vi "FT10_M4X Tester 3.vi"() -> ()   [LabVIEW 2024]
uses:
  Controls/QMH Fundamentals - Message Cluster.ctl
  <vilib>/FPGAPlugInAG/PXI-7854R/niLvFpga_Open_PXI-7854R.vi
  <vilib>/rvi/interface/common/dynamic/niFpgaDynamicAddResources.vi
  <vilib>/Utility/error.llb/Error Cluster From Error Code.vi
  <vilib>/rvi/errors/niLvFpgaAdjustHostInterfaceError.vi
  <vilib>/FPGAPlugInAG/Dynamic/niLvFpga_Close_Dynamic.vi
  <vilib>/rvi/interface/nirviOpenFPGA/nirviOpenFPGA.xnode
  FPGA Bitfiles/FT10_FPGA_7854R_Main_Rev4 BitFile.lvbitx
  FT10_FPGA_7854R_Main 4.vi
  <vilib>/rvi/interface/nirviReadWriteControl/nirviReadWriteControl.xnode
  <vilib>/rvi/interface/nirviCloseFPGA/nirviCloseFPGA.xnode
  <vilib>/rvi/interface/Simulation/niFpgaSimulationCallBeginRW.vi
  spcm_win32.dll
  NiFpgaLv.dll
panel:
  in  "Update Relays":bool
  in  "Tab Control":T1(tab)
  in  "Update Config Enum":T2(ring)
  in  "Update Config":bool
  out "Connector0/AI0":i16
  out "Connector0/AI1":i16
  out "Connector0/AI2":i16
  out "Connector0/AI3":i16
  out "Connector0/AI4":i16
  out "Connector0/AI5":i16
  out "Connector0/AI6":i16
  out "Connector0/AI7":i16
  in  "Connector0/AO0":i16
  in  "Connector0/AO2":i16
  in  "Connector0/AO3":i16
  in  "Connector0/AO4":i16
  in  "Connector0/AO5":i16
  in  "Connector0/AO6":i16
  in  "Connector0/AO1":i16
  in  "Connector0/AO7":i16
  in  "Conn0/DIO_8_15 - 75kHz":bool=TRUE
  in  "Conn0/DIO_8_15 - uSec On":u16=7
  in  "Conn0/DIO_8_15 - uSec Off":u16=6
  in  "Conn0/DIO_0_7 - uSec Off":u16=6
  in  "Conn0/DIO_0_7 - uSec On":u16=7
  in  "Conn0/DIO_0_7 - 75kHz":bool=TRUE
  in  "Conn0/DIO_8_15 In":bool[](array[boolean])=[FALSE, FALSE, FALSE, FALSE, FALSE, FALSE, FALSE, FALSE]
  in  "Conn0/DIO_0_7 In":bool[](array[boolean])=[FALSE, FALSE, FALSE, FALSE, FALSE, FALSE, FALSE, FALSE]
  out "Conn0/DIO_0_7 Out":bool[](array[boolean])
  out "Conn0/DIO_8_15 Out":bool[](array[boolean])
  in  "Conn1/DIO_32_39 - 75kHz":bool=TRUE
  in  "Conn1/DIO_32_39 - uSec On":u16=7
  in  "Conn1/DIO_32_39 - uSec Off":u16=6
  in  "Conn1/DIO_32_39 In":bool[](array[boolean])=[FALSE, FALSE, FALSE, FALSE, FALSE, FALSE, FALSE, FALSE]
  out "Conn1/DIO_32_39 Out":bool[](array[boolean])
  in  "Conn1/DIO_24_31 - 75kHz":bool=TRUE
  in  "Conn1/DIO_24_31 - uSec On":u16=7
  in  "Conn1/DIO_24_31 - uSec Off":u16=6
  in  "Conn1/DIO_16_23 - uSec Off":u16=6
  in  "Conn1/DIO_16_23 - uSec On":u16=7
  in  "Conn1/DIO_16_23 - 75kHz":bool=TRUE
  in  "Conn1/DIO_24_31 In":bool[](array[boolean])=[FALSE, FALSE, FALSE, FALSE, FALSE, FALSE, FALSE, FALSE]
  in  "Conn1/DIO_16_23 In":bool[](array[boolean])=[FALSE, FALSE, FALSE, FALSE, FALSE, FALSE, FALSE, FALSE]
  out "Conn1/DIO_16_23 Out":bool[](array[boolean])
  out "Conn1/DIO_24_31 Out":bool[](array[boolean])
  in  "Conn1/DIO_8_15 - 75kHz":bool=TRUE
  in  "Conn1/DIO_8_15 - uSec On":u16=7
  in  "Conn1/DIO_8_15 - uSec Off":u16=6
  in  "Conn1/DIO_0_7 - uSec Off":u16=6
  in  "Conn1/DIO_0_7 - uSec On":u16=7
  in  "Conn1/DIO_0_7 - 75kHz":bool=TRUE
  in  "Conn1/DIO_8_15 In":bool[](array[boolean])=[FALSE, FALSE, FALSE, FALSE, FALSE, FALSE, FALSE, FALSE]
  in  "Conn1/DIO_0_7 In":bool[](array[boolean])=[FALSE, FALSE, FALSE, FALSE, FALSE, FALSE, FALSE, FALSE]
  out "Conn1/DIO_0_7 Out":bool[](array[boolean])
  out "Conn1/DIO_8_15 Out":bool[](array[boolean])
  in  "Conn2/DIO_32_39 - 75kHz":bool=TRUE
  in  "Conn2/DIO_32_39 - uSec On":u16=7
  in  "Conn2/DIO_32_39 - uSec Off":u16=6
  in  "Conn2/DIO_32_39 In":bool[](array[boolean])=[FALSE, FALSE, FALSE, FALSE, FALSE, FALSE, FALSE, FALSE]
  out "Conn2 /DIO_32_39 Out":bool[](array[boolean])
  in  "Conn2/DIO_24_31 - 75kHz":bool=TRUE
  in  "Conn2/DIO_24_31 - uSec On":u16=7
  in  "Conn2/DIO_24_31 - uSec Off":u16=6
  in  "Conn2/DIO_16_23 - uSec Off":u16=6
  in  "Conn2/DIO_16_23 - uSec On":u16=7
  in  "Conn2/DIO_16_23 - 75kHz":bool=TRUE
  in  "Conn2/DIO_24_31 In":bool[](array[boolean])=[FALSE, FALSE, FALSE, FALSE, FALSE, FALSE, FALSE, FALSE]
  in  "Conn2/DIO_16_23 In":bool[](array[boolean])=[FALSE, FALSE, FALSE, FALSE, FALSE, FALSE, FALSE, FALSE]
  out "Conn2/DIO_16_23 Out":bool[](array[boolean])
  out "Conn2/DIO_24_31 Out":bool[](array[boolean])
  in  "Conn2/DIO_8_15 - 75kHz":bool=TRUE
  in  "Conn2/DIO_8_15 - uSec On":u16=7
  in  "Conn2/DIO_8_15 - uSec Off":u16=6
  in  "Conn2/DIO_0_7 - uSec Off":u16=6
  in  "Conn2/DIO_0_7 - uSec On":u16=7
  in  "Conn2/DIO_0_7 - 75kHz":bool=TRUE
  in  "Conn2/DIO_8_15 In":bool[](array[boolean])=[FALSE, FALSE, FALSE, FALSE, FALSE, FALSE, FALSE, FALSE]
  in  "Conn2/DIO_0_7 In":bool[](array[boolean])=[FALSE, FALSE, FALSE, FALSE, FALSE, FALSE, FALSE, FALSE]
  out "Conn2/DIO_0_7 Out":bool[](array[boolean])
  out "Conn2/DIO_8_15 Out":bool[](array[boolean])
  out "error out 2":errorcluster
  out "error out":errorcluster
  out "Array":T3(array[cluster])
  out "Waveform Array":waveform(dbl)[](graph)
  in  "stop":bool
  in  "Read":bool
  # "Conn0/DIO_0_7"
  # "Conn0/DIO_8_15"
  # "Conn0/AO_0_7"
  # "Conn0/AI0_7"
  # "Conn1/DIO_0_7"
  # "Conn1/DIO_8_15"
  # "Conn1/DIO_16_23"
  # "Conn1/DIO_24_31"
  # "Conn1/DIO_32_39"
  # "Conn2/DIO_0_7"
  # "Conn2/DIO_8_15"
  # "Conn2/DIO_16_23"
  # "Conn2/DIO_24_31"
  # "Conn2/DIO_32_39"
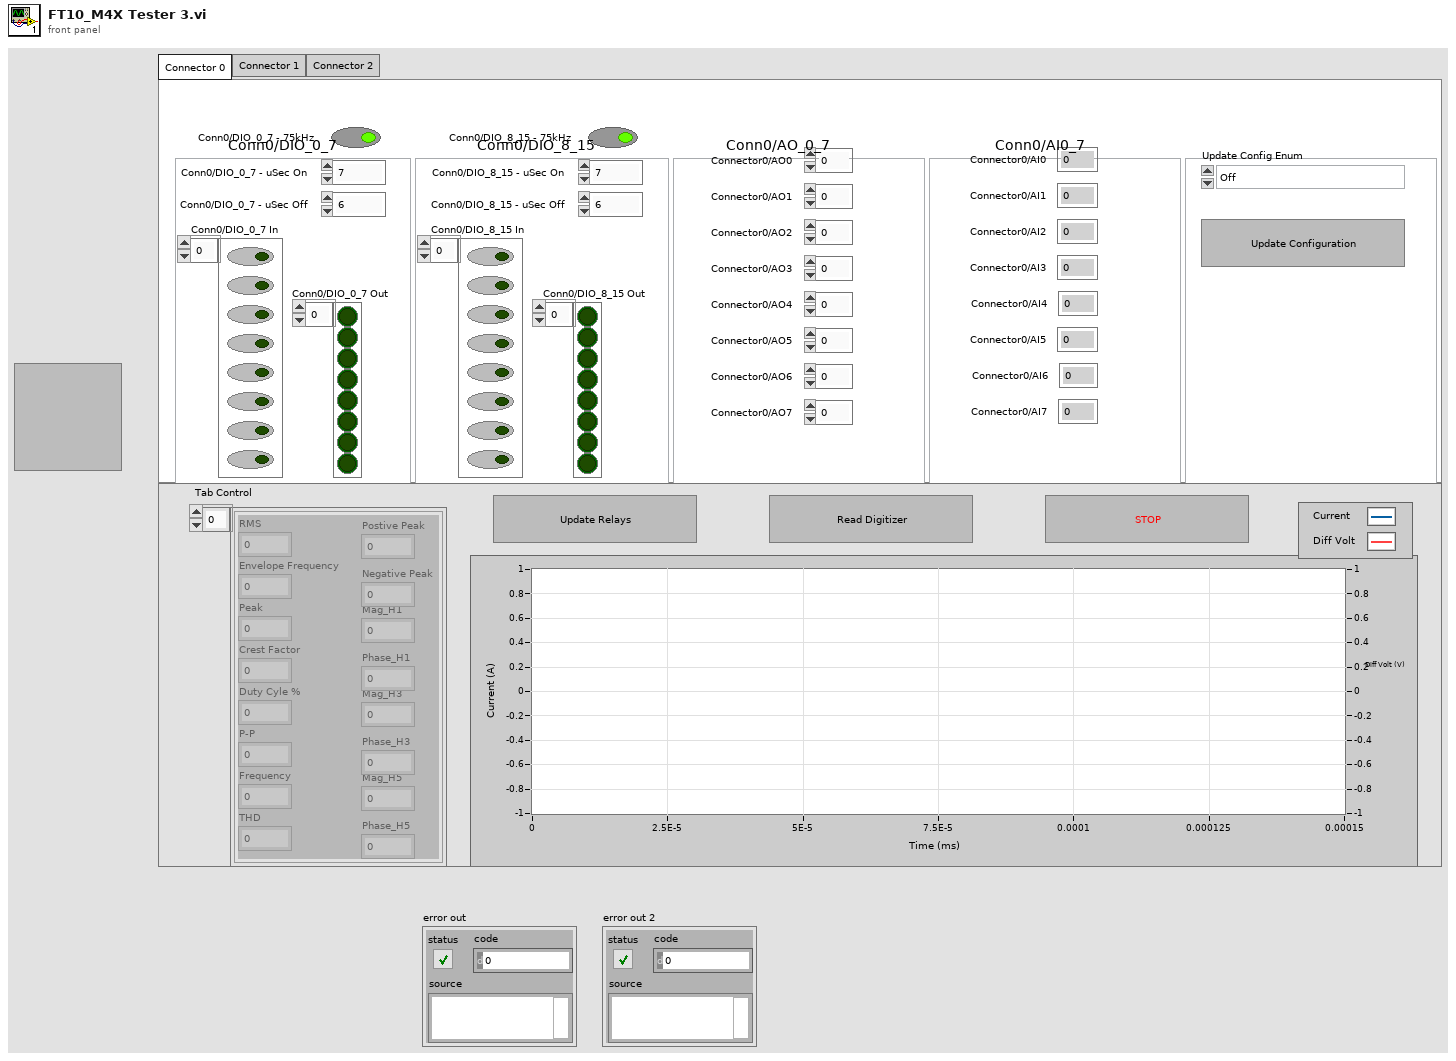
[diagram p1: front panel]
types:
  T1 = enum32{"Connector 0", "Connector 1", "Connector 2"}
  T2 = enum16{"Off", "Mono1 Relay Config", "Mono2 Relay Config", "Bipolar Relay Config", "Ligasure Relay Config", "Handswitch - Mono1 Cut", "Handswitch - Mono1 Coag", "Handswitch - Mono2 Cut", "Handswitch - Mono2 Coag", "Switch to Triverse Mode", "Switch to Mono2 - 2 button Mode", "Triverse Power 1", "Triverse Power 2", "Triverse Power 3", "Triverse Power 4", "Triverse Power 5", "Handswitch - Triverse Seal", "Handswitch - Triverse Cut", "Handswitch - Triverse Coag"}
  T3 = cluster{"RMS":dbl, "Envelope Frequency":dbl, "Peak":dbl, "Crest Factor":dbl, "Duty Cyle %":dbl, "P-P":dbl, "Frequency":dbl, "THD":dbl, "Postive Peak":dbl, "Negative Peak":dbl, "Mag_H1":dbl, "Phase_H1":dbl, "Mag_H3":dbl, "Phase_H3":dbl, "Mag_H5":dbl, "Phase_H5":dbl}[]
  T4 = typedef "QMH Fundamentals - Message Cluster.ctl" = cluster{"Message":string, "Message Data":variant}
  T5 = cluster{"Conn1/DIO_0_7 In":cluster{"Conn1/DIO_0_7 - 75kHz":bool, "Conn1/DIO_0_7 - uSec On":u16, "Conn1/DIO_0_7 In":bool[], "Conn1/DIO_0_7 - uSec Off":u16}, "Conn1/DIO_8_15 In":cluster{"Conn1/DIO_8_15 - 75kHz":bool, "Conn1/DIO_8_15 - uSec On":u16, "Conn1/DIO_8_15 In":bool[], "Conn1/DIO_8_15 - uSec Off":u16}, "Conn1/DIO_16_23 In":cluster{"Conn1/DIO_16_23 - 75kHz":bool, "Conn1/DIO_16_23 - uSec On":u16, "Conn1/DIO_16_23 In":bool[], "Conn1/DIO_16_23 - uSec Off":u16}, "Conn1/DIO_24_31 In":cluster{"Conn1/DIO_24_31 - 75kHz":bool, "Conn1/DIO_24_31 - uSec On":u16, "Conn1/DIO_24_31 In":bool[], "Conn1/DIO_24_31 - uSec Off":u16}, "Conn1/DIO_32_39 In":cluster{"Conn1/DIO_32_39 - 75kHz":bool, "Conn1/DIO_32_39 - uSec On":u16, "Conn1/DIO_32_39 In":bool[], "Conn1/DIO_32_39 - uSec Off":u16}}
  T6 = cluster{"Conn0/DIO_0_7 In":cluster{"Conn0/DIO_0_7 - 75kHz":bool, "Conn0/DIO_0_7 - uSec On":u16, "Conn0/DIO_0_7 In":bool[], "Conn0/DIO_0_7 - uSec Off":u16}, "Conn0/DIO_8_15 In":cluster{"Conn0/DIO_8_15 - 75kHz":bool, "Conn0/DIO_8_15 - uSec On":u16, "Conn0/DIO_8_15 In":bool[], "Conn0/DIO_8_15 - uSec Off":u16}}
  T7 = cluster{"Update Config":bool, "Update Config Enum":enum16{"Off", "Mono1 Relay Config", "Mono2 Relay Config", "Bipolar Relay Config", "Ligasure Relay Config", "Handswitch - Mono1 Cut", "Handswitch - Mono1 Coag", "Handswitch - Mono2 Cut", "Handswitch - Mono2 Coag", "Switch to Triverse Mode", "Switch to Mono2 - 2 button Mode", "Triverse Power 1", "Triverse Power 2", "Triverse Power 3", "Triverse Power 4", "Triverse Power 5", "Handswitch - Triverse Seal", "Handswitch - Triverse Cut", "Handswitch - Triverse Coag"}}
  T8 = cluster{"RMS":dbl, "Envelope Frequency":dbl, "Peak":dbl, "Crest Factor":dbl, "Duty Cyle %":dbl, "P-P":dbl, "Frequency":dbl, "THD":dbl, "Postive Peak":dbl, "Negative Peak":dbl, "Mag_H1":dbl, "Phase_H1":dbl, "Mag_H3":dbl, "Phase_H3":dbl, "Mag_H5":dbl, "Phase_H5":dbl}
  T9 = cluster{"Conn2/DIO_0_7 In":cluster{"Conn2/DIO_0_7 - 75kHz":bool, "Conn2/DIO_0_7 - uSec On":u16, "Conn2/DIO_0_7 In":bool[], "Conn2/DIO_0_7 - uSec Off":u16}, "Conn2/DIO_8_15 In":cluster{"Conn2/DIO_8_15 - 75kHz":bool, "Conn2/DIO_8_15 - uSec On":u16, "Conn2/DIO_8_15 In":bool[], "Conn2/DIO_8_15 - uSec Off":u16}, "Conn2/DIO_16_23 In":cluster{"Conn2/DIO_16_23 - 75kHz":bool, "Conn2/DIO_16_23 - uSec On":u16, "Conn2/DIO_16_23 In":bool[], "Conn2/DIO_16_23 - uSec Off":u16}, "Conn2/DIO_24_31 In":cluster{"Conn2/DIO_24_31 - 75kHz":bool, "Conn2/DIO_24_31 - uSec On":u16, "Conn2/DIO_24_31 In":bool[], "Conn2/DIO_24_31 - uSec Off":u16}, "Conn2/DIO_32_39 In":cluster{"Conn2/DIO_32_39 - 75kHz":bool, "Conn2/DIO_32_39 - uSec On":u16, "Conn2/DIO_32_39 In":bool[], "Conn2/DIO_32_39 - uSec Off":u16}}
  T10 = cluster{"Conn0/DIO_0_7 Out":bool[], "Conn0/DIO_8_15 Out":bool[]}
  T11 = cluster{"Conn1/DIO_0_7 Out":bool[], "Conn1/DIO_8_15 Out":bool[], "Conn1/DIO_16_23 Out":bool[], "Conn1/DIO_24_31 Out":bool[], "Conn1/DIO_32_39 Out":bool[]}
  T12 = cluster{"Conn2/DIO_0_7 Out":bool[], "Conn2/DIO_8_15 Out":bool[], "Conn2/DIO_16_23 Out":bool[], "Conn2/DIO_24_31 Out":bool[], "Conn2/DIO_32_39 Out":bool[]}
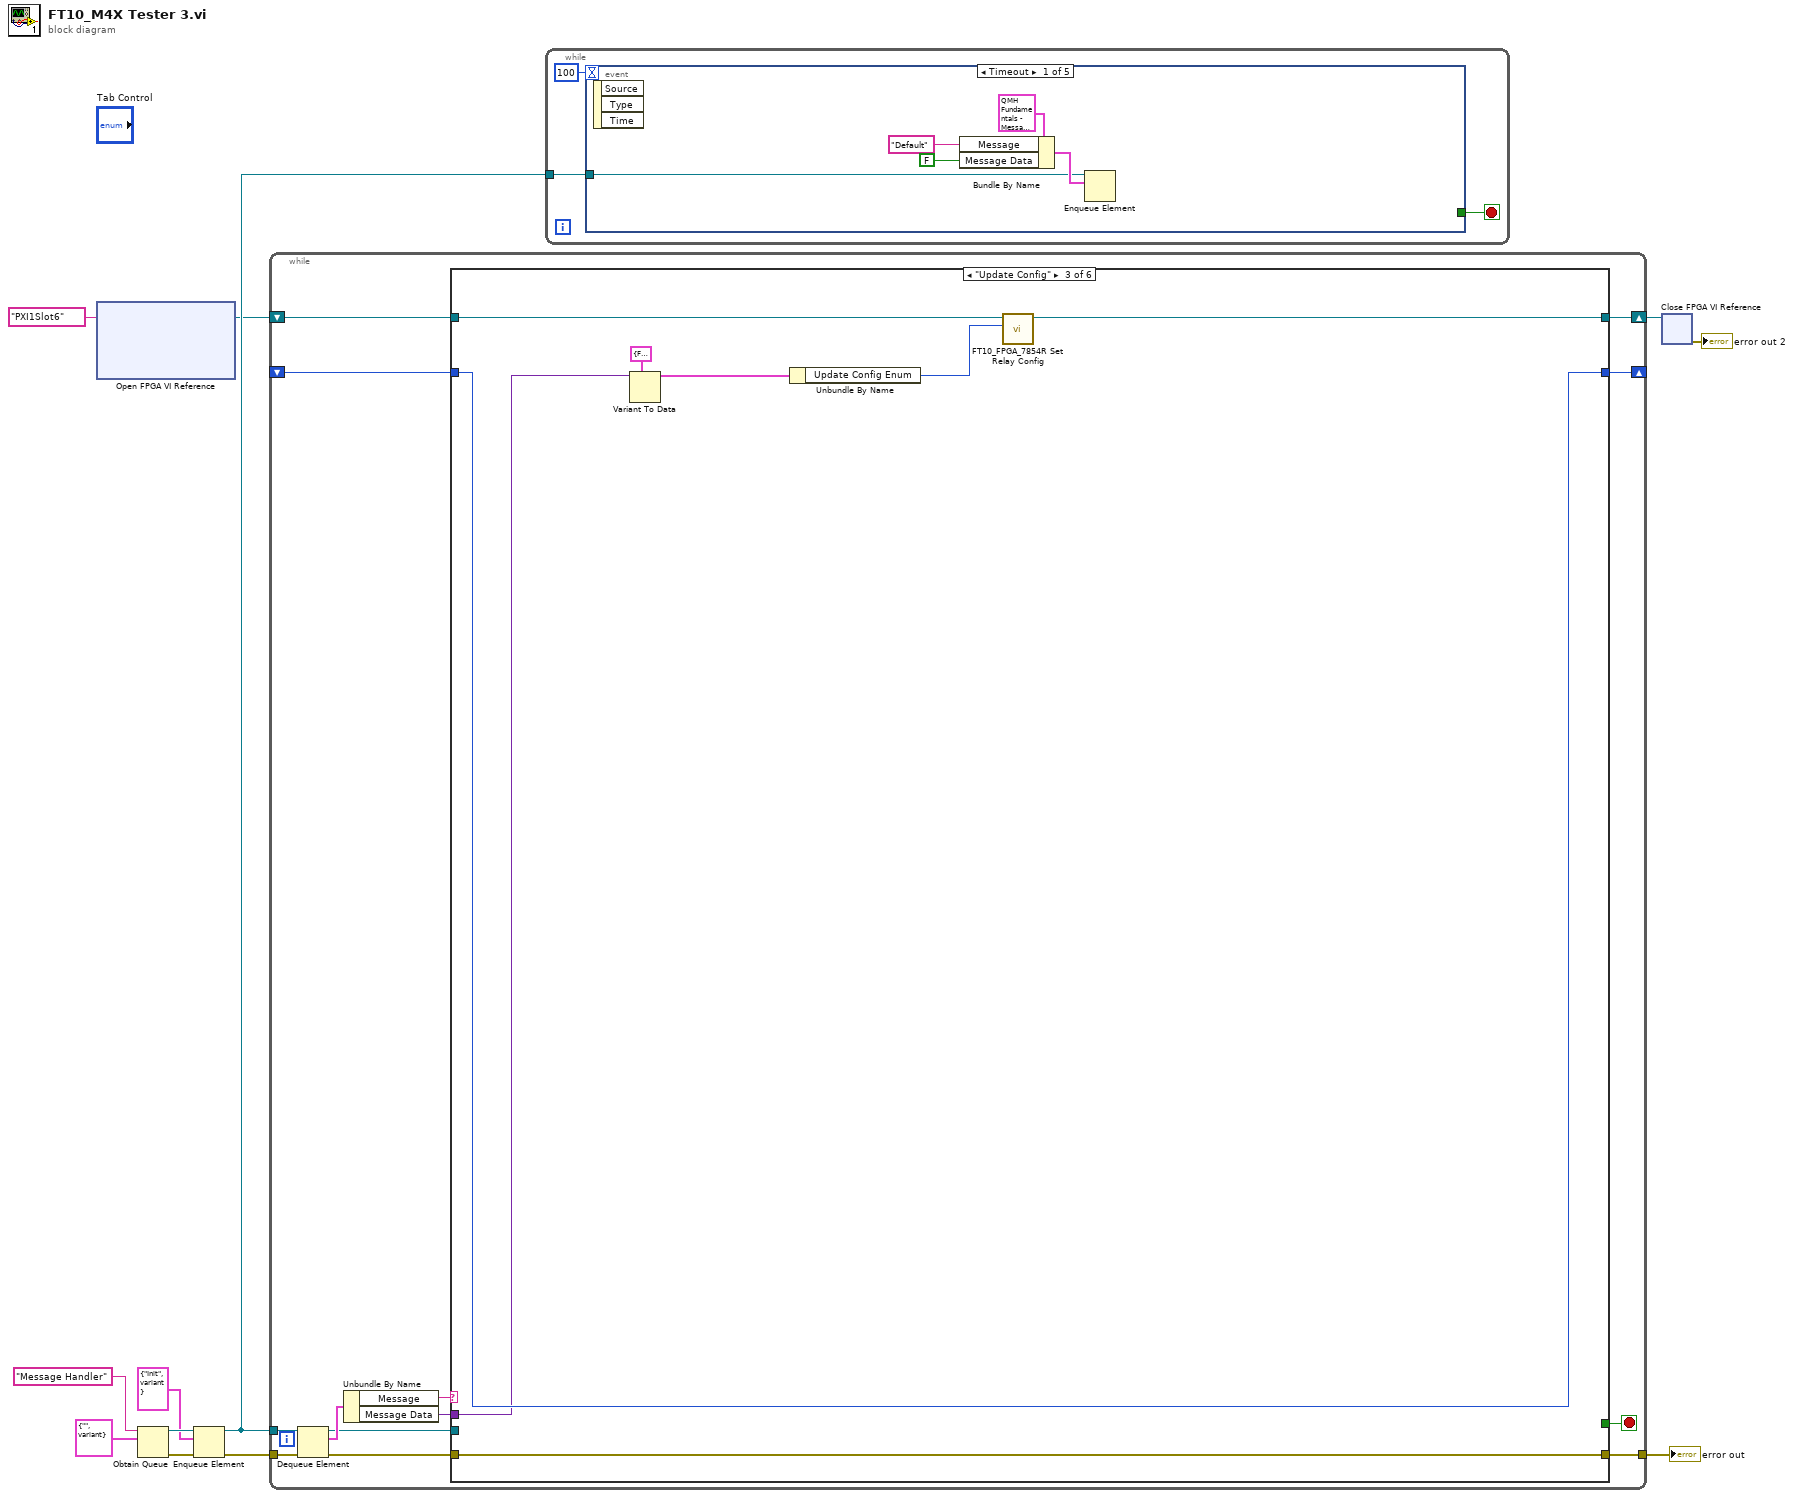
[diagram p0: block diagram]
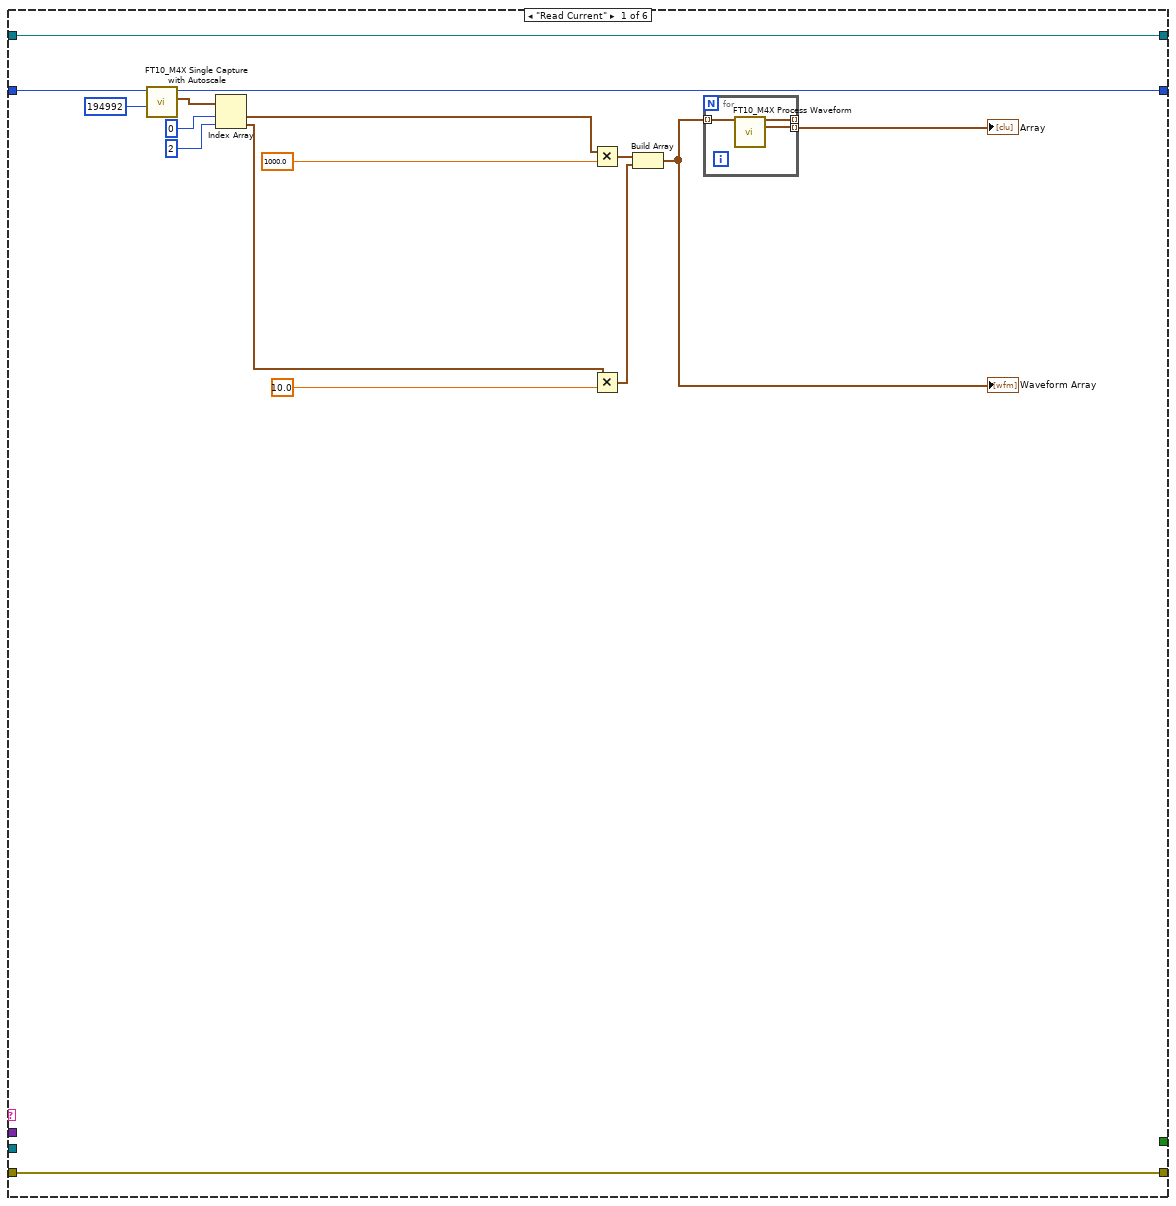
[diagram p2: hidden frame]
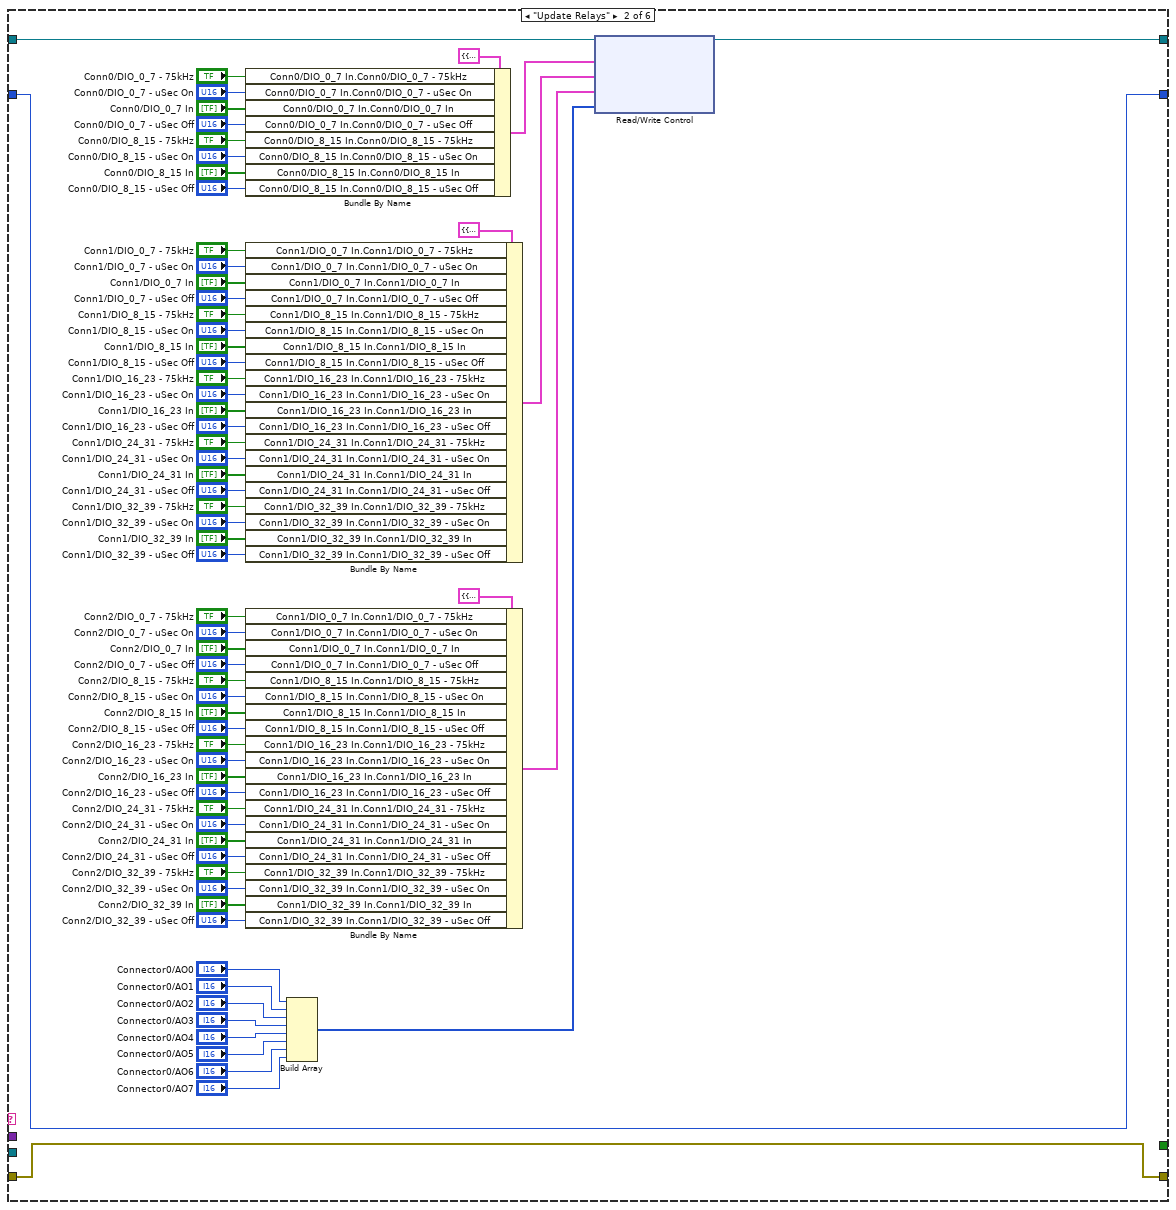
[diagram p3: hidden frame]
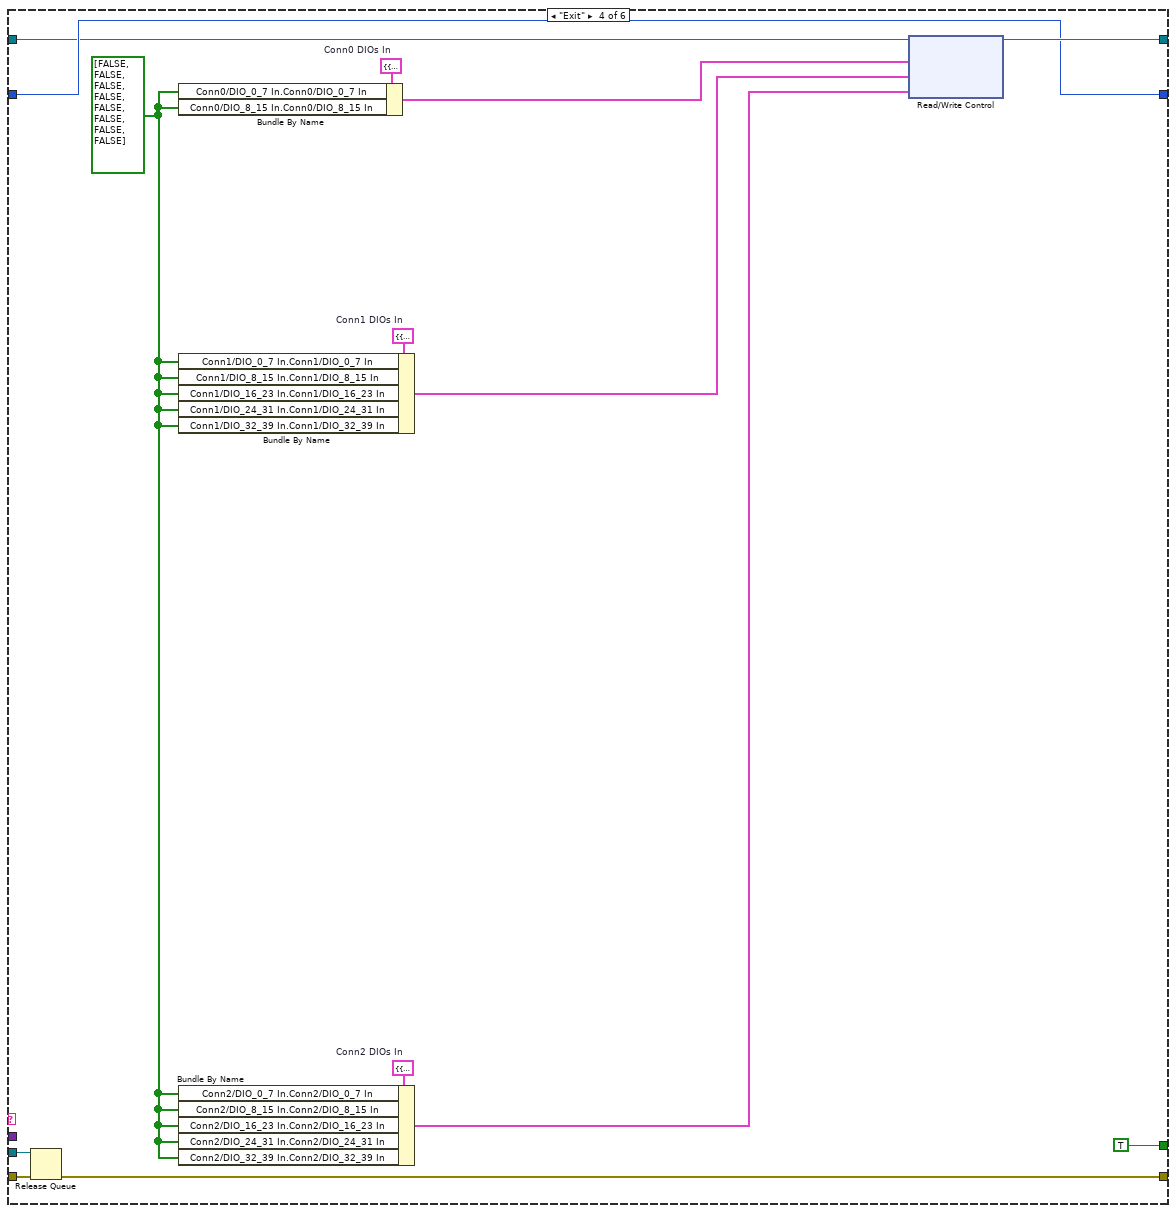
[diagram p4: hidden frame]
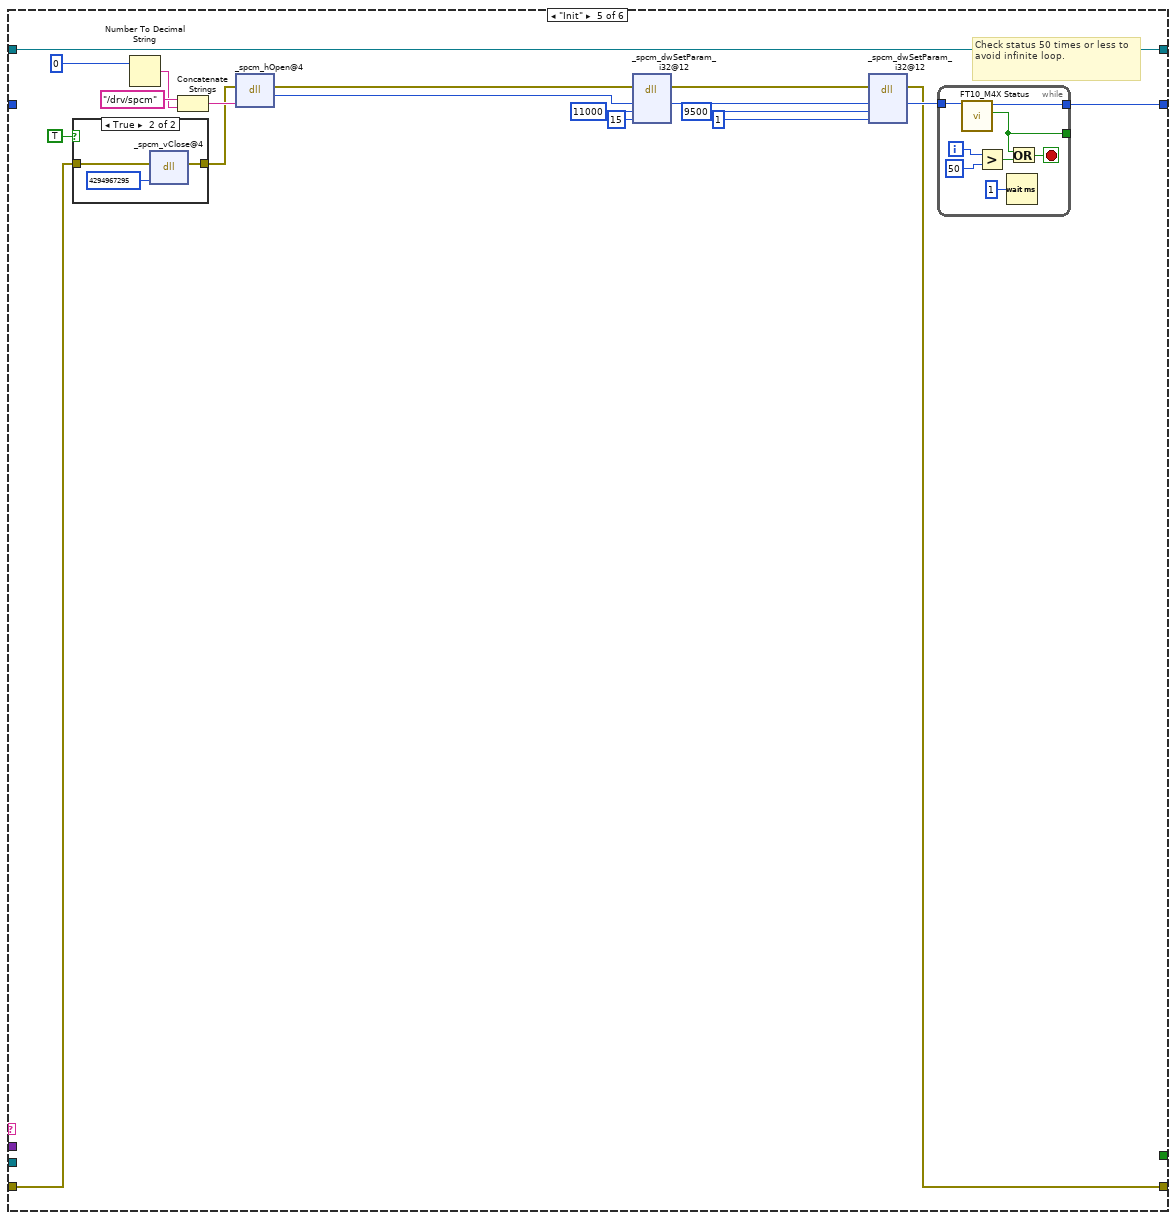
[diagram p5: hidden frame]
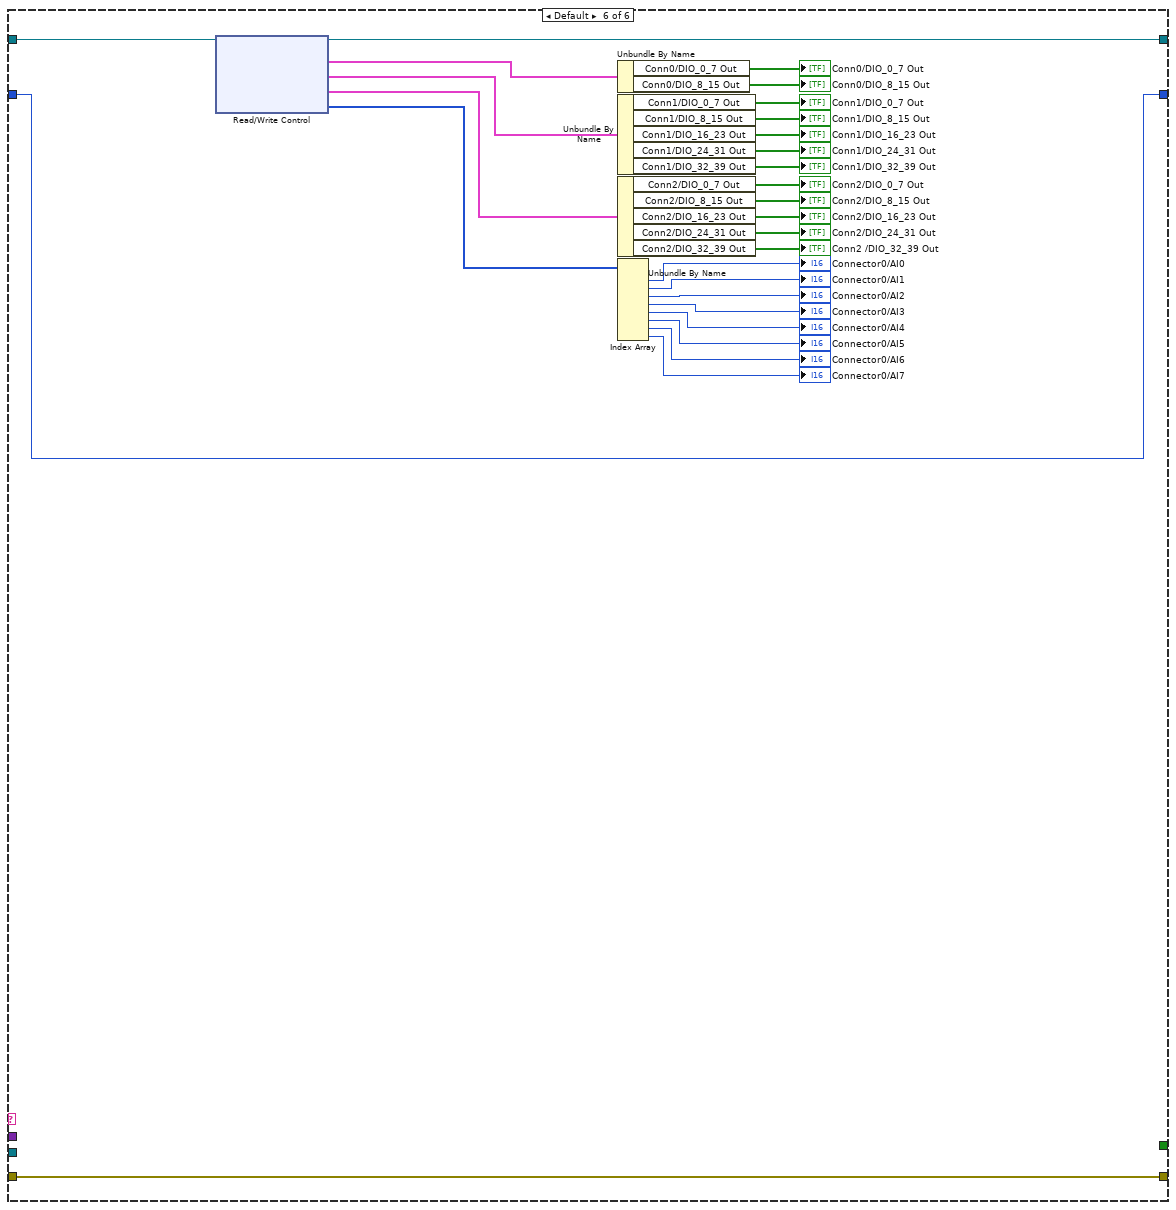
[diagram p7: hidden frame]
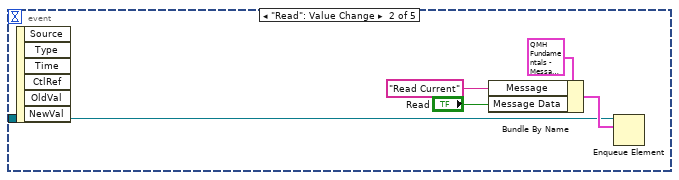
[diagram p8: hidden frame]
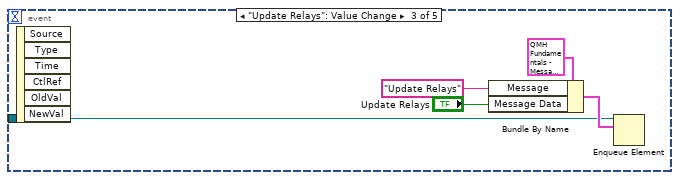
[diagram p9: hidden frame]
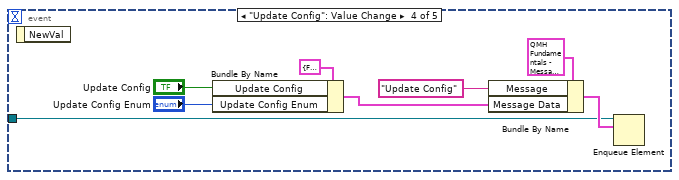
[diagram p10: hidden frame]
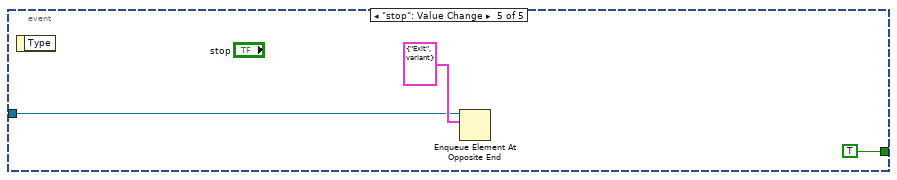
[diagram p11: hidden frame]
diagram:
  n1 = xnode "Open FPGA VI Reference"("resource name"=tag "PXI1Slot6") -> ("FPGA VI Reference Out"=w1:refnum<k20>)  [unwired: 1 in, 1 out]
  n2 = Obtain Queue(name (unnamed)="Message Handler", element data type=T4 {"Message"="", "Message Data"=variant} ("Message Cluster")) -> (queue out=w10:refnum<queue>, error out=w11:errorcluster)  [unwired: 3 in, 1 out]
  n3 = Enqueue Element(queue=w10, element=T4 {"Message"="Init", "Message Data"=variant}, error in (no error)=w11) -> (queue out=w5:refnum<queue>, error out=w7:errorcluster)  [unwired: 1 in, 1 out]
  n4 = while {
    tunnel: w5 -> [w24]
    tunnel: w7 -> [w23]
    tunnel: [w18] -> w6
    shift-right: [w17] -> _
    shift-left: _ -> [w16]
    shift-right: [w14] -> w4
    shift-left: w1 -> [w13]
    stop <- w15 stop-if-true
    n5 = Dequeue Element(queue=w24, error in (no error)=w23) -> (queue out=w22:refnum<queue>, element=w25:T4, error out=w21:errorcluster)  [unwired: 1 in, 1 out]
    n6 = Unbundle By Name(w25) -> ("Message"=w20:string, "Message Data"=w19:variant)
    n7 = case shown="\"Update Config\"" w20 {
      tunnel: w22 -> [_ _ _ w130 _ _]
      tunnel: w21 -> [w30 w108 w116 w132 w137 w192]
      tunnel: w19 -> [_ _ w114 _ _ _]
      tunnel: [w30 w108 w116 w131 w136 w192] -> w18
      tunnel: [w31 w109 w117 w128 w135 w189] -> w17
      tunnel: w16 -> [w32 w109 w117 w128 _ w189]
      tunnel: [_ _ _ TRUE _ _] -> w15
      tunnel: [w26 w110 w118 w129 w134 w190] -> w14
      tunnel: w13 -> [w26 w111 w119 w127 w134 w191]
      frame "Read Current" {
        n8 = call "FT10_M4X Single Capture with Autoscale.vi"("memsize"=194992, "Card Handle in"=w32) -> ("Data"=w35:waveform(sgl)[], "Card Handle out"=w31:u32)  [unwired: 8 in]
        n9 = Index Array(array=w35, index #1=0 ("index"), index #2=2 ("index 2")) -> (element #1=w40:waveform(sgl), element #2=w41:waveform(sgl))
        n10 = Multiply(x=w40, y=1000.0) -> (x*y=w38:waveform(dbl))
        n11 = Multiply(x=w41, y=10.0) -> (x*y=w39:waveform(dbl))
        n12 = Build Array(w38, w39) -> (w29:waveform(dbl)[])
        "Waveform Array" <- w29
        n13 = for {
          tunnel: w29 -> [w42] mode=indexing
          tunnel: [w44] -> w33 mode=indexing
          tunnel: [w43] -> _ mode=indexing
          n14 = call "FT10_M4X Process Waveform.vi"("RF Waveform In"=w42) -> ("RF Waveform Out"=w43:waveform(sgl), "Measurements"=w44:T8)  [unwired: 12 in, 1 out]
        }
        "Array" <- w33
      }
      frame "Update Relays" {
        n15 = Bundle By Name(cluster=T6 {"Conn0/DIO_0_7 In"={"Conn0/DIO_0_7 - 75kHz"=FALSE, "Conn0/DIO_0_7 - uSec On"=0, "Conn0/DIO_0_7 In"=[FALSE, FALSE, FALSE, FALSE, FALSE, FALSE, FALSE, FALSE], "Conn0/DIO_0_7 - uSec Off"=0}, "Conn0/DIO_8_15 In"={"Conn0/DIO_8_15 - 75kHz"=FALSE, "Conn0/DIO_8_15 - uSec On"=0, "Conn0/DIO_8_15 In"=[FALSE, FALSE, FALSE, FALSE, FALSE, FALSE, FALSE, FALSE], "Conn0/DIO_8_15 - uSec Off"=0}} ("Conn0 DIOs In"), "Conn0/DIO_0_7 In.Conn0/DIO_0_7 - 75kHz"="Conn0/DIO_0_7 - 75kHz", "Conn0/DIO_0_7 In.Conn0/DIO_0_7 - uSec On"="Conn0/DIO_0_7 - uSec On", "Conn0/DIO_0_7 In.Conn0/DIO_0_7 In"="Conn0/DIO_0_7 In", "Conn0/DIO_0_7 In.Conn0/DIO_0_7 - uSec Off"="Conn0/DIO_0_7 - uSec Off", "Conn0/DIO_8_15 In.Conn0/DIO_8_15 - 75kHz"="Conn0/DIO_8_15 - 75kHz", "Conn0/DIO_8_15 In.Conn0/DIO_8_15 - uSec On"="Conn0/DIO_8_15 - uSec On", "Conn0/DIO_8_15 In.Conn0/DIO_8_15 In"="Conn0/DIO_8_15 In", "Conn0/DIO_8_15 In.Conn0/DIO_8_15 - uSec Off"="Conn0/DIO_8_15 - uSec Off") -> (w98:T6)
        n16 = Bundle By Name(cluster=T5 {"Conn1/DIO_0_7 In"={"Conn1/DIO_0_7 - 75kHz"=FALSE, "Conn1/DIO_0_7 - uSec On"=0, "Conn1/DIO_0_7 In"=[FALSE, FALSE, FALSE, FALSE, FALSE, FALSE, FALSE, FALSE], "Conn1/DIO_0_7 - uSec Off"=0}, "Conn1/DIO_8_15 In"={"Conn1/DIO_8_15 - 75kHz"=FALSE, "Conn1/DIO_8_15 - uSec On"=0, "Conn1/DIO_8_15 In"=[FALSE, FALSE, FALSE, FALSE, FALSE, FALSE, FALSE, FALSE], "Conn1/DIO_8_15 - uSec Off"=0}, "Conn1/DIO_16_23 In"={"Conn1/DIO_16_23 - 75kHz"=FALSE, "Conn1/DIO_16_23 - uSec On"=0, "Conn1/DIO_16_23 In"=[FALSE, FALSE, FALSE, FALSE, FALSE, FALSE, FALSE, FALSE], "Conn1/DIO_16_23 - uSec Off"=0}, "Conn1/DIO_24_31 In"={"Conn1/DIO_24_31 - 75kHz"=FALSE, "Conn1/DIO_24_31 - uSec On"=0, "Conn1/DIO_24_31 In"=[FALSE, FALSE, FALSE, FALSE, FALSE, FALSE, FALSE, FALSE], "Conn1/DIO_24_31 - uSec Off"=0}, "Conn1/DIO_32_39 In"={"Conn1/DIO_32_39 - 75kHz"=FALSE, "Conn1/DIO_32_39 - uSec On"=0, "Conn1/DIO_32_39 In"=[FALSE, FALSE, FALSE, FALSE, FALSE, FALSE, FALSE, FALSE], "Conn1/DIO_32_39 - uSec Off"=0}} ("Conn1 DIOs In"), "Conn1/DIO_0_7 In.Conn1/DIO_0_7 - 75kHz"="Conn1/DIO_0_7 - 75kHz", "Conn1/DIO_0_7 In.Conn1/DIO_0_7 - uSec On"="Conn1/DIO_0_7 - uSec On", "Conn1/DIO_0_7 In.Conn1/DIO_0_7 In"="Conn1/DIO_0_7 In", "Conn1/DIO_0_7 In.Conn1/DIO_0_7 - uSec Off"="Conn1/DIO_0_7 - uSec Off", "Conn1/DIO_8_15 In.Conn1/DIO_8_15 - 75kHz"="Conn1/DIO_8_15 - 75kHz", "Conn1/DIO_8_15 In.Conn1/DIO_8_15 - uSec On"="Conn1/DIO_8_15 - uSec On", "Conn1/DIO_8_15 In.Conn1/DIO_8_15 In"="Conn1/DIO_8_15 In", "Conn1/DIO_8_15 In.Conn1/DIO_8_15 - uSec Off"="Conn1/DIO_8_15 - uSec Off", "Conn1/DIO_16_23 In.Conn1/DIO_16_23 - 75kHz"="Conn1/DIO_16_23 - 75kHz", "Conn1/DIO_16_23 In.Conn1/DIO_16_23 - uSec On"="Conn1/DIO_16_23 - uSec On", "Conn1/DIO_16_23 In.Conn1/DIO_16_23 In"="Conn1/DIO_16_23 In", "Conn1/DIO_16_23 In.Conn1/DIO_16_23 - uSec Off"="Conn1/DIO_16_23 - uSec Off", "Conn1/DIO_24_31 In.Conn1/DIO_24_31 - 75kHz"="Conn1/DIO_24_31 - 75kHz", "Conn1/DIO_24_31 In.Conn1/DIO_24_31 - uSec On"="Conn1/DIO_24_31 - uSec On", "Conn1/DIO_24_31 In.Conn1/DIO_24_31 In"="Conn1/DIO_24_31 In", "Conn1/DIO_24_31 In.Conn1/DIO_24_31 - uSec Off"="Conn1/DIO_24_31 - uSec Off", "Conn1/DIO_32_39 In.Conn1/DIO_32_39 - 75kHz"="Conn1/DIO_32_39 - 75kHz", "Conn1/DIO_32_39 In.Conn1/DIO_32_39 - uSec On"="Conn1/DIO_32_39 - uSec On", "Conn1/DIO_32_39 In.Conn1/DIO_32_39 In"="Conn1/DIO_32_39 In", "Conn1/DIO_32_39 In.Conn1/DIO_32_39 - uSec Off"="Conn1/DIO_32_39 - uSec Off") -> (w47:T5)
        n17 = Bundle By Name(cluster=T5 {"Conn1/DIO_0_7 In"={"Conn1/DIO_0_7 - 75kHz"=FALSE, "Conn1/DIO_0_7 - uSec On"=0, "Conn1/DIO_0_7 In"=[FALSE, FALSE, FALSE, FALSE, FALSE, FALSE, FALSE, FALSE], "Conn1/DIO_0_7 - uSec Off"=0}, "Conn1/DIO_8_15 In"={"Conn1/DIO_8_15 - 75kHz"=FALSE, "Conn1/DIO_8_15 - uSec On"=0, "Conn1/DIO_8_15 In"=[FALSE, FALSE, FALSE, FALSE, FALSE, FALSE, FALSE, FALSE], "Conn1/DIO_8_15 - uSec Off"=0}, "Conn1/DIO_16_23 In"={"Conn1/DIO_16_23 - 75kHz"=FALSE, "Conn1/DIO_16_23 - uSec On"=0, "Conn1/DIO_16_23 In"=[FALSE, FALSE, FALSE, FALSE, FALSE, FALSE, FALSE, FALSE], "Conn1/DIO_16_23 - uSec Off"=0}, "Conn1/DIO_24_31 In"={"Conn1/DIO_24_31 - 75kHz"=FALSE, "Conn1/DIO_24_31 - uSec On"=0, "Conn1/DIO_24_31 In"=[FALSE, FALSE, FALSE, FALSE, FALSE, FALSE, FALSE, FALSE], "Conn1/DIO_24_31 - uSec Off"=0}, "Conn1/DIO_32_39 In"={"Conn1/DIO_32_39 - 75kHz"=FALSE, "Conn1/DIO_32_39 - uSec On"=0, "Conn1/DIO_32_39 In"=[FALSE, FALSE, FALSE, FALSE, FALSE, FALSE, FALSE, FALSE], "Conn1/DIO_32_39 - uSec Off"=0}} ("Conn1 DIOs In"), "Conn1/DIO_0_7 In.Conn1/DIO_0_7 - 75kHz"="Conn2/DIO_0_7 - 75kHz", "Conn1/DIO_0_7 In.Conn1/DIO_0_7 - uSec On"="Conn2/DIO_0_7 - uSec On", "Conn1/DIO_0_7 In.Conn1/DIO_0_7 In"="Conn2/DIO_0_7 In", "Conn1/DIO_0_7 In.Conn1/DIO_0_7 - uSec Off"="Conn2/DIO_0_7 - uSec Off", "Conn1/DIO_8_15 In.Conn1/DIO_8_15 - 75kHz"="Conn2/DIO_8_15 - 75kHz", "Conn1/DIO_8_15 In.Conn1/DIO_8_15 - uSec On"="Conn2/DIO_8_15 - uSec On", "Conn1/DIO_8_15 In.Conn1/DIO_8_15 In"="Conn2/DIO_8_15 In", "Conn1/DIO_8_15 In.Conn1/DIO_8_15 - uSec Off"="Conn2/DIO_8_15 - uSec Off", "Conn1/DIO_16_23 In.Conn1/DIO_16_23 - 75kHz"="Conn2/DIO_16_23 - 75kHz", "Conn1/DIO_16_23 In.Conn1/DIO_16_23 - uSec On"="Conn2/DIO_16_23 - uSec On", "Conn1/DIO_16_23 In.Conn1/DIO_16_23 In"="Conn2/DIO_16_23 In", "Conn1/DIO_16_23 In.Conn1/DIO_16_23 - uSec Off"="Conn2/DIO_16_23 - uSec Off", "Conn1/DIO_24_31 In.Conn1/DIO_24_31 - 75kHz"="Conn2/DIO_24_31 - 75kHz", "Conn1/DIO_24_31 In.Conn1/DIO_24_31 - uSec On"="Conn2/DIO_24_31 - uSec On", "Conn1/DIO_24_31 In.Conn1/DIO_24_31 In"="Conn2/DIO_24_31 In", "Conn1/DIO_24_31 In.Conn1/DIO_24_31 - uSec Off"="Conn2/DIO_24_31 - uSec Off", "Conn1/DIO_32_39 In.Conn1/DIO_32_39 - 75kHz"="Conn2/DIO_32_39 - 75kHz", "Conn1/DIO_32_39 In.Conn1/DIO_32_39 - uSec On"="Conn2/DIO_32_39 - uSec On", "Conn1/DIO_32_39 In.Conn1/DIO_32_39 In"="Conn2/DIO_32_39 In", "Conn1/DIO_32_39 In.Conn1/DIO_32_39 - uSec Off"="Conn2/DIO_32_39 - uSec Off") -> (w46:T5)
        n18 = Build Array("Connector0/AO0", "Connector0/AO1", "Connector0/AO2", "Connector0/AO3", "Connector0/AO4", "Connector0/AO5", "Connector0/AO6", "Connector0/AO7") -> (w45:i16[])
        n19 = xnode "Read/Write Control"("FPGA VI Reference In"=w111, "Conn0 DIOs In"=w98, "Conn1 DIOs In"=w47, "Conn2 DIOs In"=w46, "Connector0/AO0_7"=w45) -> ("FPGA VI Reference Out"=w110:refnum<k20>)  [unwired: 1 in, 1 out]
      }
      frame "Update Config" {
        n20 = Variant To Data(type=T7 {"Update Config"=FALSE, "Update Config Enum"=enum."Triverse Power 5"}, Variant=w114) -> (data=w113:T7)  [unwired: 1 in, 1 out]
        n21 = Unbundle By Name(w113) -> ("Update Config Enum"=w112:T2)
        n22 = call "FT10_FPGA_7854R Set Relay Config.vi"("Update Config Enum"=w112, "Refnum in"=w119) -> ("Refnum out"=w118:refnum<k20>)  [unwired: 9 in]
      }
      frame "Exit" {
        w123 = T9 {"Conn2/DIO_0_7 In"={"Conn2/DIO_0_7 - 75kHz"=FALSE, "Conn2/DIO_0_7 - uSec On"=0, "Conn2/DIO_0_7 In"=[FALSE, FALSE, FALSE, FALSE, FALSE, FALSE, FALSE, FALSE], "Conn2/DIO_0_7 - uSec Off"=0}, "Conn2/DIO_8_15 In"={"Conn2/DIO_8_15 - 75kHz"=FALSE, "Conn2/DIO_8_15 - uSec On"=0, "Conn2/DIO_8_15 In"=[FALSE, FALSE, FALSE, FALSE, FALSE, FALSE, FALSE, FALSE], "Conn2/DIO_8_15 - uSec Off"=0}, "Conn2/DIO_16_23 In"={"Conn2/DIO_16_23 - 75kHz"=FALSE, "Conn2/DIO_16_23 - uSec On"=0, "Conn2/DIO_16_23 In"=[FALSE, FALSE, FALSE, FALSE, FALSE, FALSE, FALSE, FALSE], "Conn2/DIO_16_23 - uSec Off"=0}, "Conn2/DIO_24_31 In"={"Conn2/DIO_24_31 - 75kHz"=FALSE, "Conn2/DIO_24_31 - uSec On"=0, "Conn2/DIO_24_31 In"=[FALSE, FALSE, FALSE, FALSE, FALSE, FALSE, FALSE, FALSE], "Conn2/DIO_24_31 - uSec Off"=0}, "Conn2/DIO_32_39 In"={"Conn2/DIO_32_39 - 75kHz"=FALSE, "Conn2/DIO_32_39 - uSec On"=0, "Conn2/DIO_32_39 In"=[FALSE, FALSE, FALSE, FALSE, FALSE, FALSE, FALSE, FALSE], "Conn2/DIO_32_39 - uSec Off"=0}}  # Conn2 DIOs In
        w124 = T5 {"Conn1/DIO_0_7 In"={"Conn1/DIO_0_7 - 75kHz"=FALSE, "Conn1/DIO_0_7 - uSec On"=0, "Conn1/DIO_0_7 In"=[FALSE, FALSE, FALSE, FALSE, FALSE, FALSE, FALSE, FALSE], "Conn1/DIO_0_7 - uSec Off"=0}, "Conn1/DIO_8_15 In"={"Conn1/DIO_8_15 - 75kHz"=FALSE, "Conn1/DIO_8_15 - uSec On"=0, "Conn1/DIO_8_15 In"=[FALSE, FALSE, FALSE, FALSE, FALSE, FALSE, FALSE, FALSE], "Conn1/DIO_8_15 - uSec Off"=0}, "Conn1/DIO_16_23 In"={"Conn1/DIO_16_23 - 75kHz"=FALSE, "Conn1/DIO_16_23 - uSec On"=0, "Conn1/DIO_16_23 In"=[FALSE, FALSE, FALSE, FALSE, FALSE, FALSE, FALSE, FALSE], "Conn1/DIO_16_23 - uSec Off"=0}, "Conn1/DIO_24_31 In"={"Conn1/DIO_24_31 - 75kHz"=FALSE, "Conn1/DIO_24_31 - uSec On"=0, "Conn1/DIO_24_31 In"=[FALSE, FALSE, FALSE, FALSE, FALSE, FALSE, FALSE, FALSE], "Conn1/DIO_24_31 - uSec Off"=0}, "Conn1/DIO_32_39 In"={"Conn1/DIO_32_39 - 75kHz"=FALSE, "Conn1/DIO_32_39 - uSec On"=0, "Conn1/DIO_32_39 In"=[FALSE, FALSE, FALSE, FALSE, FALSE, FALSE, FALSE, FALSE], "Conn1/DIO_32_39 - uSec Off"=0}}  # Conn1 DIOs In
        w126 = T6 {"Conn0/DIO_0_7 In"={"Conn0/DIO_0_7 - 75kHz"=FALSE, "Conn0/DIO_0_7 - uSec On"=0, "Conn0/DIO_0_7 In"=[FALSE, FALSE, FALSE, FALSE, FALSE, FALSE, FALSE, FALSE], "Conn0/DIO_0_7 - uSec Off"=0}, "Conn0/DIO_8_15 In"={"Conn0/DIO_8_15 - 75kHz"=FALSE, "Conn0/DIO_8_15 - uSec On"=0, "Conn0/DIO_8_15 In"=[FALSE, FALSE, FALSE, FALSE, FALSE, FALSE, FALSE, FALSE], "Conn0/DIO_8_15 - uSec Off"=0}}  # Conn0 DIOs In
        w122 = bool[] [FALSE, FALSE, FALSE, FALSE, FALSE, FALSE, FALSE, FALSE] ("Conn1/DIO_0_7 In")
        n23 = Release Queue(queue=w130, error in (no error)=w132) -> (error out=w131:errorcluster)  [unwired: 1 in, 2 out]
        n24 = Bundle By Name(cluster=w126, "Conn0/DIO_0_7 In.Conn0/DIO_0_7 In"=w122, "Conn0/DIO_8_15 In.Conn0/DIO_8_15 In"=w122) -> (w125:T6)
        n25 = Bundle By Name(cluster=w124, "Conn1/DIO_0_7 In.Conn1/DIO_0_7 In"=w122, "Conn1/DIO_8_15 In.Conn1/DIO_8_15 In"=w122, "Conn1/DIO_16_23 In.Conn1/DIO_16_23 In"=w122, "Conn1/DIO_24_31 In.Conn1/DIO_24_31 In"=w122, "Conn1/DIO_32_39 In.Conn1/DIO_32_39 In"=w122) -> (w121:T5)
        n26 = Bundle By Name(cluster=w123, "Conn2/DIO_0_7 In.Conn2/DIO_0_7 In"=w122, "Conn2/DIO_8_15 In.Conn2/DIO_8_15 In"=w122, "Conn2/DIO_16_23 In.Conn2/DIO_16_23 In"=w122, "Conn2/DIO_24_31 In.Conn2/DIO_24_31 In"=w122, "Conn2/DIO_32_39 In.Conn2/DIO_32_39 In"=w122) -> (w120:T9)
        n27 = xnode "Read/Write Control"("FPGA VI Reference In"=w127, "Conn0 DIOs In"=w125, "Conn1 DIOs In"=w121, "Conn2 DIOs In"=w120) -> ("FPGA VI Reference Out"=w129:refnum<k20>)  [unwired: 1 in, 1 out]
      }
      frame "Init" {
        # "Check status 50 times or less to avoid infinite loop."
        n28 = case shown="True" TRUE ("reset device") {
          tunnel: w137 -> [w161 w164]
          tunnel: [w161 w163] -> w147
          frame False {
          }
          frame True {
            n29 = dll-call lib="spcm_win32.dll" fn="_spcm_vClose@4"(error in=w164, "hDrv"=u32 4294967295) -> (error out=w163:errorcluster)  [unwired: 4 in, 1 out]
          }
        }
        n30 = Number To Decimal String(number=u32 0 ("Board #")) -> (decimal integer string=w148:string)  [unwired: 1 in]
        n31 = Concatenate Strings("/drv/spcm" ("szDeviceName"), w148) -> (w149:string)
        n32 = dll-call lib="spcm_win32.dll" fn="_spcm_hOpen@4"(error in=w147, "szDeviceName"=w149) -> (error out=w145:errorcluster, "hDrv"=w144:u32)  [unwired: 3 in, 1 out]
        n33 = dll-call lib="spcm_win32.dll" fn="_spcm_dwSetParam_i32@12" label="SPC_CHENABLE"(error in=w145, "hDrv"=w144, "lRegister"=11000, "lValue"=15) -> (error out=w141:errorcluster, "hDrv"=w140:u32)  [unwired: 5 in, 1 out]
        n34 = dll-call lib="spcm_win32.dll" fn="_spcm_dwSetParam_i32@12" label="SPC_CARDMODE"(error in=w141, "hDrv"=w140, "lRegister"=9500, "lValue"=1) -> (error out=w136:errorcluster, "hDrv"=w152:u32)  [unwired: 5 in, 1 out]
        n35 = while {
          tunnel: w152 -> [w159]
          tunnel: [w158] -> w135
          tunnel: [w153] -> _
          i -> [w157]
          stop <- w155 stop-if-true
          n36 = call "FT10_M4X Status.vi"("Card Handle in"=w159) -> ("Ready?"=w153:bool, "Card Handle out"=w158:u32)  [unwired: 9 in]
          n37 = Greater?(x=w157, y=50) -> (0:w154:bool)
          n38 = Wait (ms)(milliseconds to wait=u32 1) -> ()  [unwired: 1 out]
          n39 = Or(x=w153, y=w154) -> (x .or. y?=w155:bool)
        }
      }
      frame Default {
        n40 = xnode "Read/Write Control"("FPGA VI Reference In"=w191) -> ("FPGA VI Reference Out"=w190:refnum<k20>, "Conn0 - DIOs Out"=w168:T10, "Conn1 - DIOs Out"=w167:T11, "Conn2 - DIOs Out"=w166:T12, "Connector0/AI0"=w165:i16[])  [unwired: 1 in, 1 out]
        n41 = Unbundle By Name(w168) -> ("Conn0/DIO_0_7 Out"=→"Conn0/DIO_0_7 Out":bool[], "Conn0/DIO_8_15 Out"=→"Conn0/DIO_8_15 Out":bool[])
        n42 = Unbundle By Name(w167) -> ("Conn1/DIO_0_7 Out"=→"Conn1/DIO_0_7 Out":bool[], "Conn1/DIO_8_15 Out"=→"Conn1/DIO_8_15 Out":bool[], "Conn1/DIO_16_23 Out"=→"Conn1/DIO_16_23 Out":bool[], "Conn1/DIO_24_31 Out"=→"Conn1/DIO_24_31 Out":bool[], "Conn1/DIO_32_39 Out"=→"Conn1/DIO_32_39 Out":bool[])
        n43 = Unbundle By Name(w166) -> ("Conn2/DIO_0_7 Out"=→"Conn2/DIO_0_7 Out":bool[], "Conn2/DIO_8_15 Out"=→"Conn2/DIO_8_15 Out":bool[], "Conn2/DIO_16_23 Out"=→"Conn2/DIO_16_23 Out":bool[], "Conn2/DIO_24_31 Out"=→"Conn2/DIO_24_31 Out":bool[], "Conn2/DIO_32_39 Out"=→"Conn2 /DIO_32_39 Out":bool[])
        n44 = Index Array(array=w165) -> (element #1=→"Connector0/AI0":i16, element #2=→"Connector0/AI1":i16, element #3=→"Connector0/AI2":i16, element #4=→"Connector0/AI3":i16, element #5=→"Connector0/AI4":i16, element #6=→"Connector0/AI5":i16, element #7=→"Connector0/AI6":i16, element #8=→"Connector0/AI7":i16)  [unwired: 8 in]
      }
    }
  }
  "error out" <- w6
  n45 = while {
    tunnel: w5 -> [w195]
    stop <- w194 stop-if-true
    n46 = event shown="[0] Timeout" {
      selector: _ -> [_ _ _ _ _]
      dyn-events: _ -> [_ _ _ _ _]
      timeout: 100 -> [_ _ _ _ _]
      tunnel: w195 -> [w196 w202 w207 w215 w220]
      tunnel: [_ _ _ _ TRUE] -> w194
      event Timeout {
        n47 = event-data() -> ()  [unwired: 1 in, 3 out]
        n48 = Bundle By Name(cluster=T4 {"Message"="Fornax Connect/Disconnect", "Message Data"=variant} ("element"), "Message"="Default", "Message Data"=FALSE ("Update Relays 2")) -> (w198:T4)
        n49 = Enqueue Element(queue=w196, element=w198) -> ()  [unwired: 2 in, 3 out]
      }
      event "Read": Value Change {
        n50 = event-data() -> ()  [unwired: 1 in, 6 out]
        n51 = Bundle By Name(cluster=T4 {"Message"="Fornax Connect/Disconnect", "Message Data"=variant} ("element"), "Message"="Read Current", "Message Data"="Read") -> (w203:T4)
        n52 = Enqueue Element(queue=w202, element=w203) -> ()  [unwired: 2 in, 3 out]
      }
      event "Update Relays": Value Change {
        n53 = event-data() -> ()  [unwired: 1 in, 6 out]
        n54 = Bundle By Name(cluster=T4 {"Message"="Fornax Connect/Disconnect", "Message Data"=variant} ("element"), "Message"="Update Relays", "Message Data"="Update Relays") -> (w208:T4)
        n55 = Enqueue Element(queue=w207, element=w208) -> ()  [unwired: 2 in, 3 out]
      }
      event "Update Config": Value Change {
        n56 = event-data() -> ()  [unwired: 1 in, 1 out]
        n57 = Bundle By Name(cluster=T7 {"Update Config"=FALSE, "Update Config Enum"=enum."Triverse Power 5"}, "Update Config"="Update Config", "Update Config Enum"="Update Config Enum") -> (w213:T7)
        n58 = Bundle By Name(cluster=T4 {"Message"="Fornax Connect/Disconnect", "Message Data"=variant} ("element"), "Message"="Update Config", "Message Data"=w213) -> (w216:T4)
        n59 = Enqueue Element(queue=w215, element=w216) -> ()  [unwired: 2 in, 3 out]
      }
      event "stop": Value Change {
        n60 = event-data() -> ()  [unwired: 1 in, 1 out]
        n61 = Enqueue Element At Opposite End(queue=w220, element=T4 {"Message"="Exit", "Message Data"=variant}) -> ()  [unwired: 2 in, 3 out]
      }
    }
  }
  n62 = xnode "Close FPGA VI Reference"("FPGA VI Reference In"=w4) -> ("error out"=→"error out 2":errorcluster)  [unwired: 1 in]
